vi "FPGA SPI_Read Write.vi"(7 "Total Bits":u16=8, 8 "error in":errorcluster, 9 "Write Data":u8[](array[numeric]), 10 "Port":i8, 11 "FPGA VI Reference":T1) -> (0 "error out":errorcluster, 2 "Read Data":u8[](array[numeric]), 3 "FPGA VI Reference Out":T1)   [LabVIEW 2014]
uses:
  Controls/FPGA Reference.ctl
  FPGA/SPI/Controls/FPGA SPI_FPGA SPI State.ctl
  <vilib>/Utility/error.llb/Error Cluster From Error Code.vi
  <vilib>/rvi/errors/niLvFpgaAdjustHostInterfaceError.vi
  <vilib>/rvi/interface/nirviReadWriteControl/nirviReadWriteControl.xnode
  FPGA Bitfiles/FormulaElectric2_FPGATarget_FPGA_KFopRbsiCjk.lvbitx
  FPGA/Sensor Library/FPGA.vi
  NiFpgaLv.dll
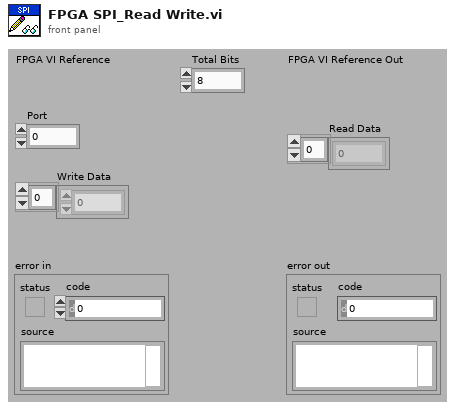
[diagram p1: front panel]
types:
  T1 = typedef "FPGA Reference.ctl" = refnum<k20>
  T2 = enum16{"Start", "Write", "Read", "Wait Until Done"}
  T3 = typedef "FPGA SPI_FPGA SPI State.ctl" = enum8{"Idle", "Read/Write SPI", "Configure"}
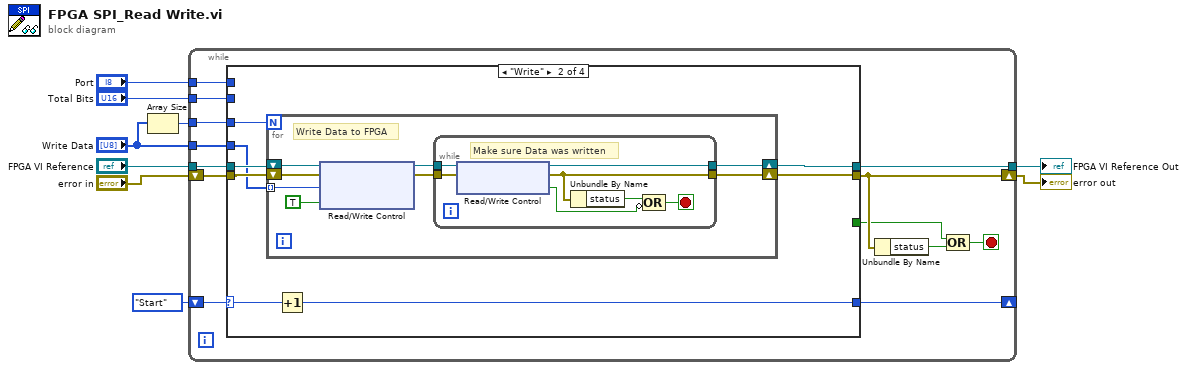
[diagram p0: block diagram]
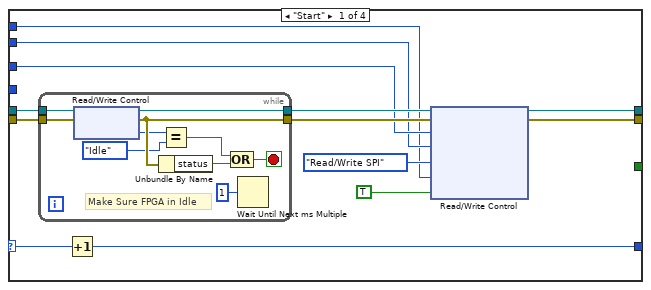
[diagram p2: hidden frame]
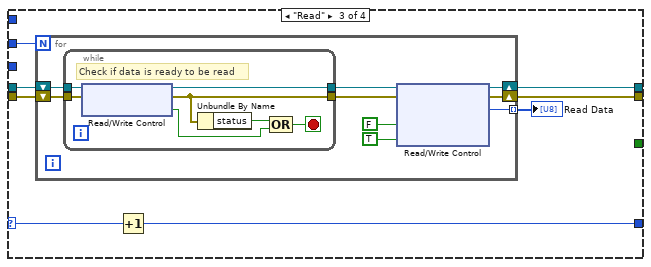
[diagram p3: hidden frame]
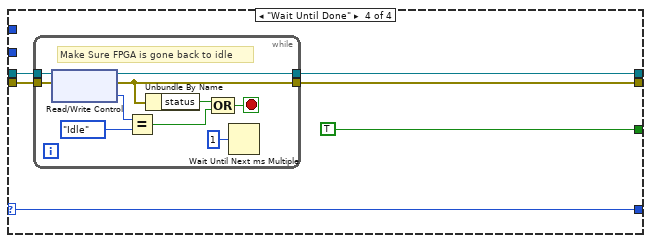
[diagram p4: hidden frame]
diagram:
  n1 = Array Size(array="Write Data") -> (size(s)=w8:i32)
  n2 = while {
    tunnel: "FPGA VI Reference" -> [w22]
    tunnel: w8 -> [w20]
    tunnel: "Write Data" -> [w19]
    tunnel: [w18] -> w6
    shift-right: [w17] -> w5
    shift-left: "error in" -> [w21]
    shift-right: [w12] -> _
    shift-left: T2."Start" -> [w13]
    tunnel: "Total Bits" -> [w11]
    tunnel: "Port" -> [w10]
    stop <- w14 stop-if-true
    n3 = case shown="\"Write\"" w13 {
      selector: w13 -> [w24 w46 w70 w94]
      tunnel: w22 -> [w33 w53 w75 w98]
      tunnel: w21 -> [w32 w52 w74 w97]
      tunnel: w20 -> [w31 w51 w73 _]
      tunnel: w19 -> [_ w50 _ _]
      tunnel: [w29 w48 w72 w96] -> w18
      tunnel: [w30 w49 w71 w95] -> w17
      tunnel: [_ _ _ TRUE] -> w16
      tunnel: [w23 w47 w69 w94] -> w12
      tunnel: w11 -> [w27 _ _ _]
      tunnel: w10 -> [w25 _ _ _]
      frame "Start" {
        n4 = while {
          tunnel: w33 -> [w45]
          tunnel: [w44] -> w35
          tunnel: w32 -> [w43]
          tunnel: [w40] -> w34
          stop <- w41 stop-if-true
          # "Make Sure FPGA in Idle"
          n5 = xnode "Read/Write Control"("FPGA VI Reference In"=w45, "error in"=w43) -> ("FPGA VI Reference Out"=w44:T1, "error out"=w40:errorcluster, "SPI_Cmd"=w37:T3)
          n6 = Unbundle By Name(w40) -> ("status"=w42:bool)
          n7 = Equal?(x=w37, y=FPGA_SPI_FPGA_SPI_State."Idle" ("Type")) -> (x = y?=w38:bool)
          n8 = Compound Arithmetic op=OR(w38, w42) -> (w41:bool)
          n9 = Wait Until Next ms Multiple(millisecond multiple=u32 1) -> ()  [unwired: 1 out]
        }
        n10 = Increment(x=w24) -> (x+1=w23:T2)
        n11 = xnode "Read/Write Control"("FPGA VI Reference In"=w35, "error in"=w34, "SPI_Total Bytes"=w31, "SPI_Total Bits"=w27, "SPI_Cmd"=FPGA_SPI_FPGA_SPI_State."Read/Write SPI" ("Cmd"), "SPI_Port"=w25, "SPI_Start"=TRUE ("Start")) -> ("FPGA VI Reference Out"=w29:T1, "error out"=w30:errorcluster)
      }
      frame "Write" {
        n12 = for {
          N: w51 -> [_]
          shift-right: [w55] -> w48
          shift-left: w53 -> [w61]
          shift-right: [w54] -> w49
          shift-left: w52 -> [w60]
          tunnel: w50 -> [w57] mode=indexing
          # "Write Data to FPGA"
          n13 = xnode "Read/Write Control"("FPGA VI Reference In"=w61, "error in"=w60, "SPI_Write Data"=w57, "SPI_Write Flag"=TRUE ("Write Flag")) -> ("FPGA VI Reference Out"=w59:T1, "error out"=w58:errorcluster)
          n14 = while {
            tunnel: w59 -> [w68]
            tunnel: w58 -> [w67]
            tunnel: [w66] -> w55
            tunnel: [w65] -> w54
            stop <- w62 stop-if-true
            # "Make sure Data was written"
            n15 = xnode "Read/Write Control"("FPGA VI Reference In"=w68, "error in"=w67) -> ("FPGA VI Reference Out"=w66:T1, "error out"=w65:errorcluster, "SPI_Write Flag"=w63:bool)
            n16 = Unbundle By Name(w65) -> ("status"=w64:bool)
            n17 = Compound Arithmetic op=OR(w64, invert w63) -> (w62:bool)
          }
        }
        n18 = Increment(x=w46) -> (x+1=w47:T2)
      }
      frame "Read" {
        n19 = for {
          N: w73 -> [_]
          shift-right: [w81] -> w72
          shift-left: w75 -> [w85]
          shift-right: [w80] -> w71
          shift-left: w74 -> [w84]
          tunnel: [w79] -> w76 mode=indexing
          n20 = while {
            tunnel: w85 -> [w87]
            tunnel: w84 -> [w92]
            tunnel: [w91] -> w83
            tunnel: [w90] -> w82
            stop <- w88 stop-if-true
            # "Check if data is ready to be read"
            n21 = xnode "Read/Write Control"("FPGA VI Reference In"=w87, "error in"=w92) -> ("FPGA VI Reference Out"=w91:T1, "error out"=w90:errorcluster, "SPI_Read Flag"=w86:bool)
            n22 = Unbundle By Name(w90) -> ("status"=w89:bool)
            n23 = Compound Arithmetic op=OR(w89, w86) -> (w88:bool)
          }
          n24 = xnode "Read/Write Control"("FPGA VI Reference In"=w83, "error in"=w82, "SPI_Read Flag"=FALSE ("Read Flag"), "SPI_Ack Read"=TRUE ("Write Flag")) -> ("FPGA VI Reference Out"=w81:T1, "error out"=w80:errorcluster, "SPI_Read Data"=w79:u8)
        }
        "Read Data" <- w76
        n25 = Increment(x=w70) -> (x+1=w69:T2)
      }
      frame "Wait Until Done" {
        n26 = while {
          tunnel: w98 -> [w108]
          tunnel: [w107] -> w96
          tunnel: w97 -> [w106]
          tunnel: [w103] -> w95
          stop <- w100 stop-if-true
          # "Make Sure FPGA is gone back to idle"
          n27 = xnode "Read/Write Control"("FPGA VI Reference In"=w108, "error in"=w106) -> ("FPGA VI Reference Out"=w107:T1, "error out"=w103:errorcluster, "SPI_Cmd"=w105:T3)
          n28 = Equal?(x=w105, y=FPGA_SPI_FPGA_SPI_State."Idle") -> (x = y?=w101:bool)
          n29 = Unbundle By Name(w103) -> ("status"=w102:bool)
          n30 = Compound Arithmetic op=OR(w102, w101) -> (w100:bool)
          n31 = Wait Until Next ms Multiple(millisecond multiple=u32 1) -> ()  [unwired: 1 out]
        }
      }
    }
    n32 = Unbundle By Name(w17) -> ("status"=w15:bool)
    n33 = Compound Arithmetic op=OR(w16, w15) -> (w14:bool)
  }
  "FPGA VI Reference Out" <- w6
  "error out" <- w5
